vi "SubVi to read from file.vi"(8 "error in (no error)":errorcluster, 10 "section":string, 11 "Refnum in":T1) -> (0 "error out":errorcluster, 2 "Results":u32[](array[numeric]), 3 "Refnum out":T1)   [LabVIEW 2020]
uses:
  <vilib>/Utility/config.llb/Config Data RefNum.ctl
  <vilib>/Utility/config.llb/Read Key (U32).vi
  <vilib>/Utility/config.llb/NI_LVConfig.lvlib
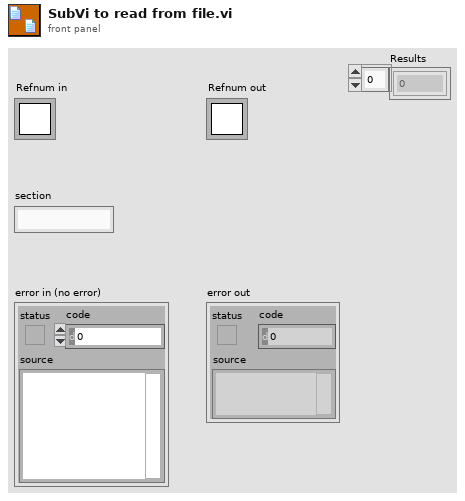
[diagram p1: front panel]
types:
  T1 = typedef "NI_LVConfig.lvlib/Config Data RefNum.ctl" = refnum<k1>
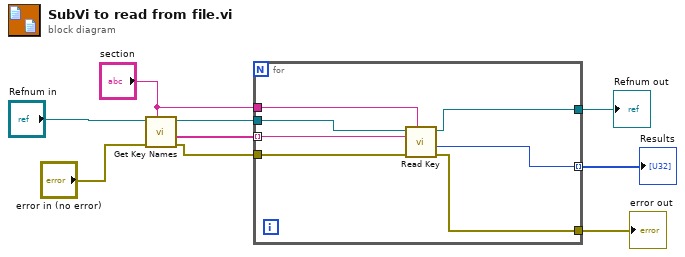
[diagram p0: block diagram]
diagram:
  n1 = call <vilib>:"Get Key Names.vi"("section"="section", "error in (no error)"="error in (no error)", "refnum"="Refnum in") -> ("error out"=w7:errorcluster, "key names"=w4:string[], "refnum out"=w6:T1)  [unwired: 5 in, 1 out]
  n2 = for {
    tunnel: w4 -> [w16] mode=indexing
    tunnel: "section" -> [w15]
    tunnel: w6 -> [w14]
    tunnel: w7 -> [w13]
    tunnel: [w12] -> w8
    tunnel: [w11] -> w1 mode=indexing
    tunnel: [w10] -> w9
    n3 = call-poly <vilib>:"Read Key.vi"("section"=w15, "error in (no error)"=w13, "key"=w16, "refnum"=w14) -> ("error out"=w10:errorcluster, "value"=w11:u32, "refnum out"=w12:T1)  [unwired: 4 in, 1 out]
  }
  "Refnum out" <- w8
  "error out" <- w9
  "Results" <- w1
